vi "Add Email Attachment.vi"(8 "error in (no error)":errorcluster, 10 "Attachment Path":path=path "E:/LabVIEW相关/研究所培训计划/FirstDay/Demo1/src/Demo4/1. 视觉采集工具包的使用.vi", 11 "StmpEmail in":refnum<class "StmpEmail.lvclass">) -> (0 "error out":errorcluster, 3 "StmpEmail out":refnum<class "StmpEmail.lvclass">)   [LabVIEW 2015, in "StmpEmail.lvclass"]
uses:
  StmpEmail.lvclass
  StmpEmail.lvclass/StmpEmail.ctl
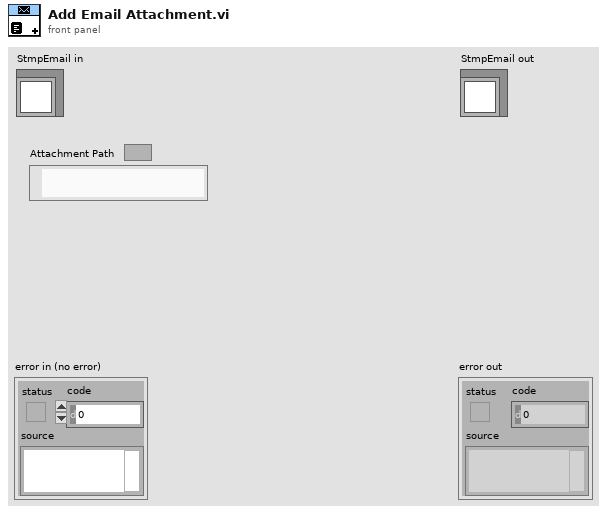
[diagram p1: front panel]
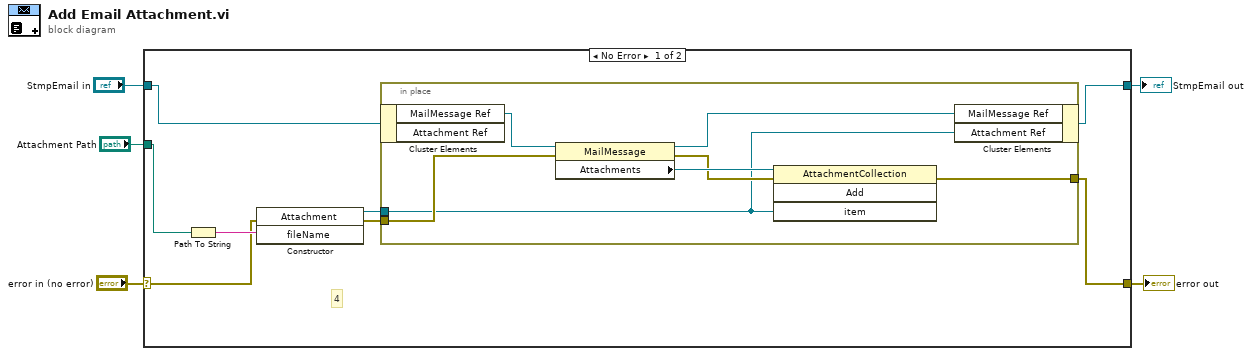
[diagram p0: block diagram]
diagram:
  n1 = case shown="No Error" "error in (no error)" {
    selector: "error in (no error)" -> [w9 w22]
    tunnel: [w6 w22] -> w4
    tunnel: [w7 w21] -> w2
    tunnel: "StmpEmail in" -> [w11 w21]
    tunnel: "Attachment Path" -> [w13 _]
    frame No Error {
      # "4"
      n2 = Path To String(path=w13) -> (string=w12:string)
      n3 = constructor class="Attachment"(error in=w9, "fileName"=w12) -> (reference out=w10:refnum<k24>, error out=w8:errorcluster)  [unwired: 2 in, 2 out]
      n4 = in-place {
        in-place-border: w10 -> [w14]
        in-place-border: w8 -> [w18]
        in-place-border: [w15] -> w6
        n5 = in-place-cluster #1(w11) -> ("MailMessage Ref"=w20:refnum<k24>)  [unwired: 1 out]
        n6 = property class="MailMessage"(reference=w20, error in=w18) -> (reference out=w16:refnum<k24>, error out=w17:errorcluster, "Attachments"=w19:refnum<k24>)
        n7 = invoke class="AttachmentCollection" method="Add"(reference=w19, error in=w17, "item"=w14) -> (error out=w15:errorcluster)  [unwired: 1 in, 3 out]
        n8 = in-place-cluster #1("MailMessage Ref"=w16, "Attachment Ref"=w14) -> (w7:refnum<class "StmpEmail.lvclass">)
      }
    }
    frame Error {
    }
  }
  "error out" <- w4
  "StmpEmail out" <- w2
